vi "toJSON.vi"(8 "error in (no error)":errorcluster, 11 "tBSONBoolean in":refnum<class "tBSONBoolean.lvclass">) -> (0 "error out":errorcluster, 2 "JSON":string, 3 "tBSONBoolean out":refnum<class "tBSONBoolean.lvclass">)   [LabVIEW 2013, in "BSON.lvlib" / "tBSONBoolean.lvclass"]
uses:
  tBSONBoolean.lvclass
  tBSONElement/tBSONElement.lvclass
  getValue.vi
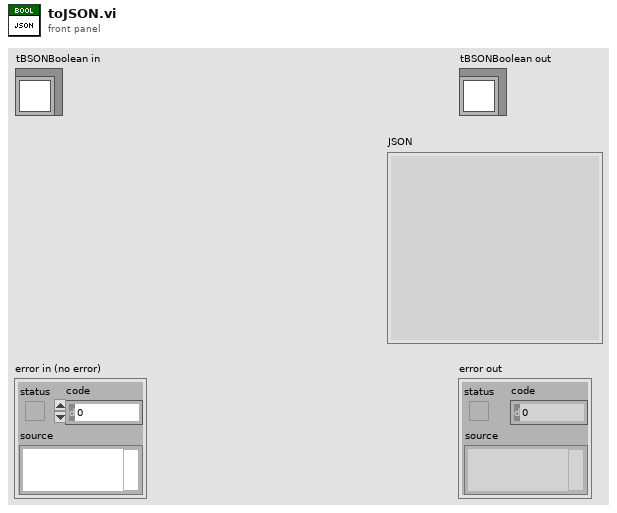
[diagram p1: front panel]
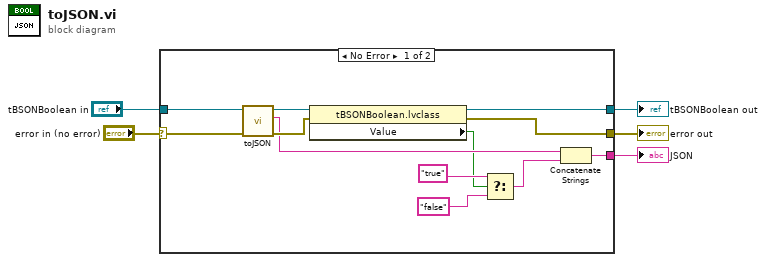
[diagram p0: block diagram]
diagram:
  n1 = case shown="No Error" "error in (no error)" {
    selector: "error in (no error)" -> [w15 w18]
    tunnel: "tBSONBoolean in" -> [w17 w19]
    tunnel: [w14 w19] -> w3
    tunnel: [w7 _] -> w2
    tunnel: [w6 w18] -> w1
    frame No Error {
      n2 = call-parent "toJSON.vi"("error in (no error)"=w15, "tBSONElement in"=w17) -> ("error out"=w13:errorcluster, "JSON"=w12:string, "tBSONElement out"=w16:refnum<class "tBSONBoolean.lvclass">)  [unwired: 7 in]
      n3 = property class="tBSONBoolean.lvclass"(reference=w16, error in=w13) -> (reference out=w14:refnum<class "tBSONBoolean.lvclass">, error out=w6:errorcluster, "Value"=w8:bool)
      n4 = Select(t="true", s=w8, f="false") -> (s? t:f=w11:string)
      n5 = Concatenate Strings(w12, w11) -> (w7:string)
    }
    frame Error {
    }
  }
  "error out" <- w1
  "tBSONBoolean out" <- w3
  "JSON" <- w2
